vi "Deconfigure Cameras.vi"(8 "error in (no error)":errorcluster, 11 "Gantry Class in":refnum<class "Gantry Class.lvclass">) -> (0 "error out":errorcluster, 3 "Gantry Class out":refnum<class "Gantry Class.lvclass">)   [LabVIEW 2011, in "Gantry Class.lvclass"]
uses:
  Gantry Class.lvclass
  <vilib>/userdefined/High Color/IMAQdx.ctl
  <vilib>/vision/driver/NI_Vision_Acquisition_Software.lvlib
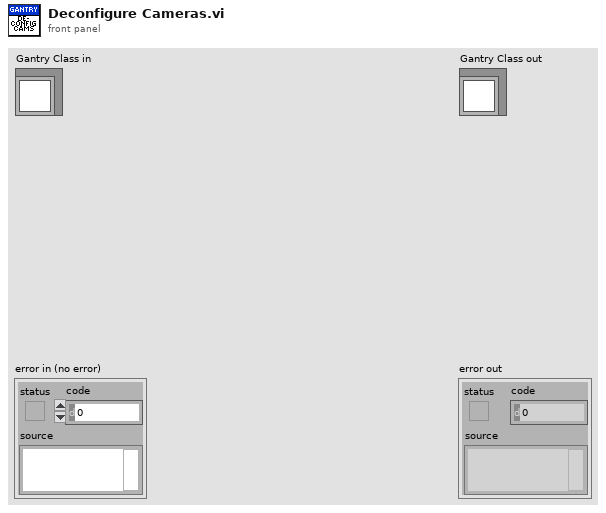
[diagram p1: front panel]
types:
  T1 = typedef "IMAQdx.ctl" = refnum<k21>
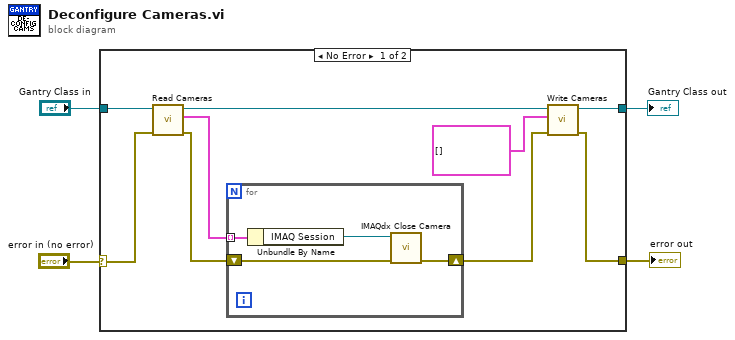
[diagram p0: block diagram]
diagram:
  n1 = case shown="No Error" "error in (no error)" {
    selector: "error in (no error)" -> [w9 w19]
    tunnel: [w11 w19] -> w3
    tunnel: [w13 w18] -> w1
    tunnel: "Gantry Class in" -> [w10 w18]
    frame No Error {
      n2 = call-dynamic "Read Cameras.vi"("error in (no error)"=w9, "Gantry Class in"=w10) -> ("error out"=w7:errorcluster, "Cameras"=w8:cluster{"Name":string, "IMAQ Session":T1}[], "Gantry Class out"=w6:refnum<class "Gantry Class.lvclass">)  [unwired: 7 in]
      n3 = for {
        tunnel: w8 -> [w17] mode=indexing
        shift-right: [w14] -> w12
        shift-left: w7 -> [w15]
        n4 = Unbundle By Name(w17) -> ("IMAQ Session"=w16:T1)
        n5 = call <vilib>:"IMAQdx Close Camera.vi"("error in"=w15, "Session In"=w16) -> ("error out"=w14:errorcluster)  [unwired: 9 in]
      }
      n6 = call-dynamic "Write Cameras.vi"("error in (no error)"=w12, "Cameras"=cluster{"Name":string, "IMAQ Session":T1}[] [], "Gantry Class in"=w6) -> ("error out"=w11:errorcluster, "Gantry Class out"=w13:refnum<class "Gantry Class.lvclass">)  [unwired: 7 in]
    }
    frame Error {
    }
  }
  "error out" <- w3
  "Gantry Class out" <- w1
